vi "Get Bitfile Path from NIVS.vi"(8 "error in (no error)":errorcluster, 11 "ID in":T1 format="%.0x") -> (0 "error out":errorcluster, 1 "Path":string, 3 "ID out":T1 format="%.0x")   [LabVIEW 2011, in "Engine Sim System Explorer.lvlib"]
uses:
  Engine Sim System Explorer.lvlib
  <vilib>/NI Veristand/Custom Device API/Custom Device Item Ref.ctl
  NationalInstruments.VeriStand.SystemDefinitionAPI
  <vilib>/Utility/sysdir.llb/System Directory Type.ctl
  <vilib>/NI Veristand/Custom Device Offline API/Custom Device Offline API.lvlib
  <vilib>/NI Veristand/Custom Device API/Custom Device API.lvlib
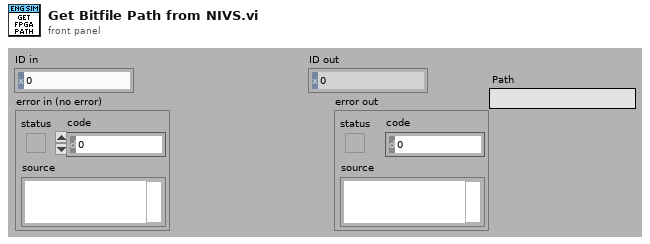
[diagram p1: front panel]
types:
  T1 = typedef "Custom Device API.lvlib/Custom Device Item Ref.ctl" = u64
  T2 = typedef "System Directory Type.ctl" = i32
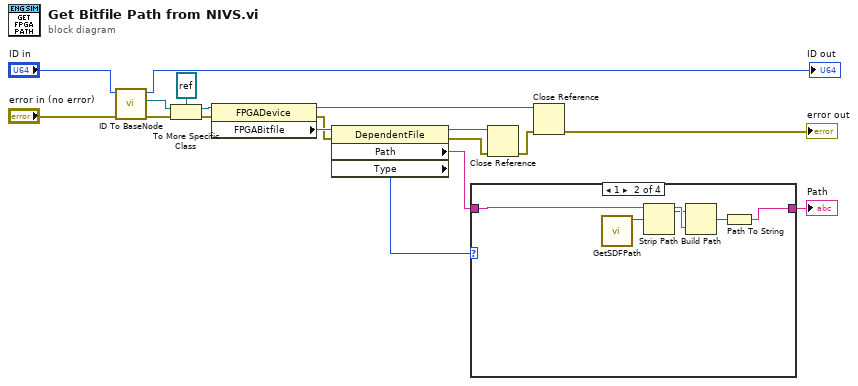
[diagram p0: block diagram]
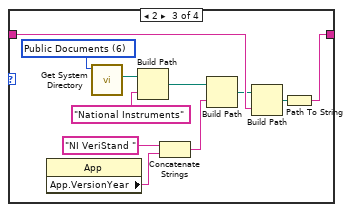
[diagram p3: hidden frame]
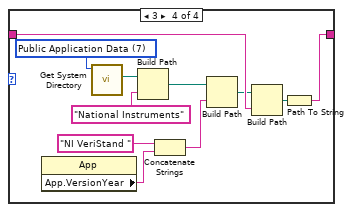
[diagram p4: hidden frame]
diagram:
  n1 = call <vilib>:"ID To BaseNode.vi"("error in (no error)"="error in (no error)", "ID in"="ID in") -> ("error out"=w16:errorcluster, "BaseNode"=w18:refnum<k24>, "ID out"=→"ID out":u64)  [unwired: 7 in]
  n2 = To More Specific Class(target class=refnum<k24> refnum ("BaseNodeType"), reference=w18, error in=w16) -> (specific class reference=w15:refnum<k24>, error out=w14:errorcluster)
  n3 = property class="FPGADevice"(reference=w15, error in=w14) -> (reference out=w9:refnum<k24>, error out=w7:errorcluster, "FPGABitfile"=w8:refnum<k24>)
  n4 = property class="DependentFile"(reference=w8, error in=w7) -> (reference out=w5:refnum<k24>, error out=w6:errorcluster, "Path"=w1:string, "Type"=w3:i32)
  n5 = case shown="1" w3 {
    tunnel: [w19 w22 w30 w41] -> w2
    tunnel: w1 -> [w19 w24 w32 w43]
    frame 0, Default {
    }
    frame 1 {
      n6 = call "GetSDFPath.vi"() -> ("SDF File Path"=w21:path)  [unwired: 10 in, 1 out]
      n7 = Strip Path(path=w21) -> (stripped path=w20:path)  [unwired: 1 out]
      n8 = Build Path(base path=w20, name or relative path=w24) -> (appended path=w23:path)
      n9 = Path To String(path=w23) -> (string=w22:string)
    }
    frame 2 {
      w35 = T2 6 items=["User Home"=0, "User Desktop"=1, "User Documents"=2, "User Application Data"=3, "User Preferences"=4, "User Temporary"=5, "Public Documents"=6, "Public Application Data"=7, "Public Preferences"=8, "Public Cache"=13, "System Core Libraries"=9, "System Installed Libraries"=10, "Application Files"=11, "Boot Volume Root"=12] ("system directory type")
      n10 = property class="App"() -> ("App.VersionYear"=w26:string)  [unwired: 2 in, 2 out]
      n11 = call <vilib>:"Get System Directory.vi"("system directory type"=w35) -> ("system directory"=w34:path)  [unwired: 10 in]
      n12 = Build Path(base path=w34, name or relative path="National Instruments") -> (appended path=w28:path)
      n13 = Concatenate Strings("NI VeriStand " ("name or relative path"), w26) -> (w25:string)
      n14 = Build Path(base path=w28, name or relative path=w25) -> (appended path=w29:path)
      n15 = Build Path(base path=w29, name or relative path=w32) -> (appended path=w31:path)
      n16 = Path To String(path=w31) -> (string=w30:string)
    }
    frame 3 {
      w46 = T2 7 items=["User Home"=0, "User Desktop"=1, "User Documents"=2, "User Application Data"=3, "User Preferences"=4, "User Temporary"=5, "Public Documents"=6, "Public Application Data"=7, "Public Preferences"=8, "Public Cache"=13, "System Core Libraries"=9, "System Installed Libraries"=10, "Application Files"=11, "Boot Volume Root"=12] ("system directory type")
      n17 = property class="App"() -> ("App.VersionYear"=w37:string)  [unwired: 2 in, 2 out]
      n18 = call <vilib>:"Get System Directory.vi"("system directory type"=w46) -> ("system directory"=w45:path)  [unwired: 10 in]
      n19 = Build Path(base path=w45, name or relative path="National Instruments") -> (appended path=w39:path)
      n20 = Concatenate Strings("NI VeriStand " ("name or relative path"), w37) -> (w36:string)
      n21 = Build Path(base path=w39, name or relative path=w36) -> (appended path=w40:path)
      n22 = Build Path(base path=w40, name or relative path=w43) -> (appended path=w42:path)
      n23 = Path To String(path=w42) -> (string=w41:string)
    }
  }
  "Path" <- w2
  n24 = Close Reference(reference=w5, error in (no error)=w6) -> (error out=w4:errorcluster)
  n25 = Close Reference(reference=w9, error in (no error)=w4) -> (error out=→"error out":errorcluster)
